vi "Tree_GetAllDescendants.vi"(8 "Error In":errorcluster, 10 "Tag":string, 11 "Tree Refnum IN":refnum<vi>) -> (0 "Error Out":errorcluster, 2 "All Descendants":string[](array[string]), 3 "Tree Refnum OUT":refnum<vi>)   [LabVIEW 2012]
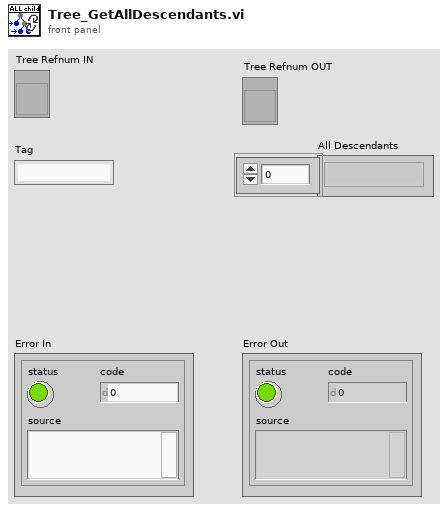
[diagram p1: front panel]
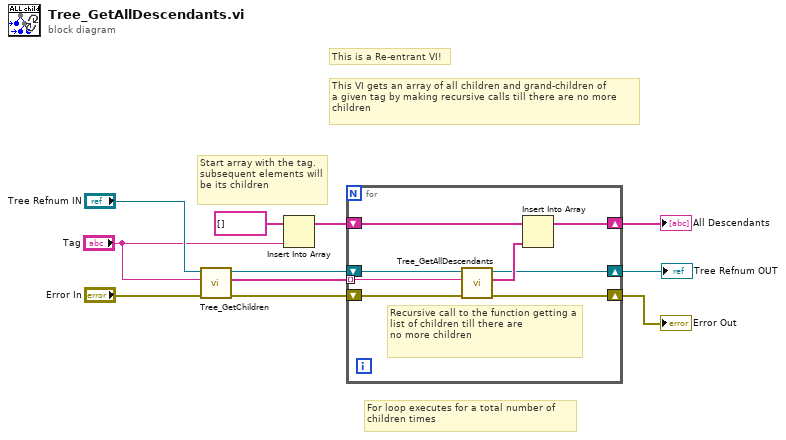
[diagram p0: block diagram]
diagram:
  # "For loop executes for a total number of \nchildren times"
  # "Start array with the tag.\nsubsequent elements will be its children"
  # "This VI gets an array of all children and grand-children of\na given tag by making recursive calls till there are no more\nchildren"
  # "This is a Re-entrant VI!"
  n1 = call "Tree_GetChildren.vi"("Error In"="Error In", "Parent Tag"="Tag", "Tree Refnum IN"="Tree Refnum IN") -> ("Error Out"=w2:errorcluster, "Children Tags"=w6:string[], "Tree Refnum OUT"=w10:refnum<vi>)  [unwired: 6 in]
  n2 = Insert Into Array(array=string[] [], new element="Tag") -> (w3:string[])  [unwired: 1 in]
  n3 = for {
    tunnel: w6 -> [w19] mode=indexing
    shift-right: [w15] -> w8
    shift-left: w3 -> [w14]
    shift-right: [w16] -> w7
    shift-left: w2 -> [w17]
    shift-right: [w12] -> w1
    shift-left: w10 -> [w18]
    # "Recursive call to the function getting a list of children till there are\nno more children"
    n4 = call "Tree_GetAllDescendants.vi"("Error In"=w17, "Tag"=w19, "Tree Refnum IN"=w18) -> ("Error Out"=w16:errorcluster, "All Descendants"=w13:string[], "Tree Refnum OUT"=w12:refnum<vi>)  [unwired: 6 in]
    n5 = Insert Into Array(array=w14, new element=w13) -> (w15:string[])  [unwired: 1 in]
  }
  "Error Out" <- w7
  "All Descendants" <- w8
  "Tree Refnum OUT" <- w1
